vi "Range.vi"(1 "Array":dbl[](array[numeric])) -> (0 "Range":dbl)   [LabVIEW 2020]
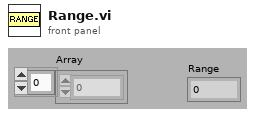
[diagram p1: front panel]
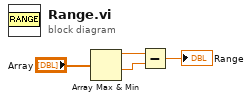
[diagram p0: block diagram]
diagram:
  n1 = Array Max & Min(array="Array") -> (max value=w3:dbl, min value=w2:dbl)  [unwired: 2 out]
  n2 = Subtract(x=w3, y=w2) -> (x-y=→"Range":dbl)
